vi "Robotic Arm controler.vi"(1 "write?":bool, 2 "Servo angle":dbl(knob)=90.0 scale=0.0..180.0, 3 "Servo number":i32(knob)=3 scale=1.0..6.0) -> (0 "Command to robotic arm":string)   [LabVIEW 2015]
doc: "Sends the commands to the Robotic Arm based on the servo number and angle provided as the inputs."
uses:
  <vilib>/Instr/_visa.llb/VISA Configure Serial Port (Instr).vi
panel:
  # "Servo number"
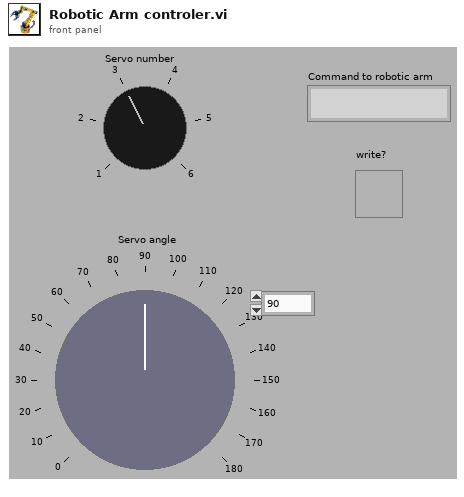
[diagram p1: front panel]
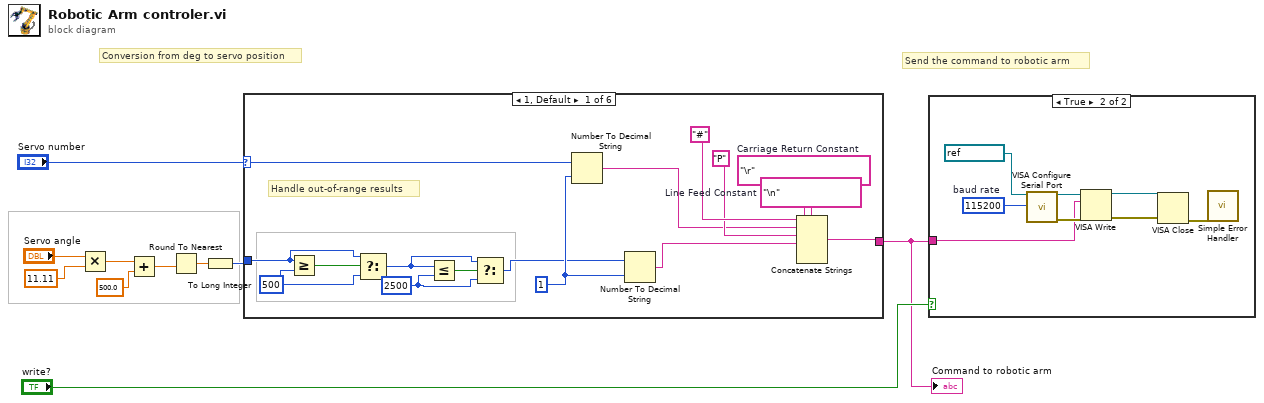
[diagram p0: block diagram]
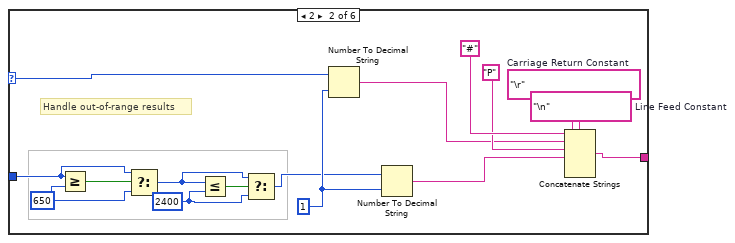
[diagram p3: hidden frame]
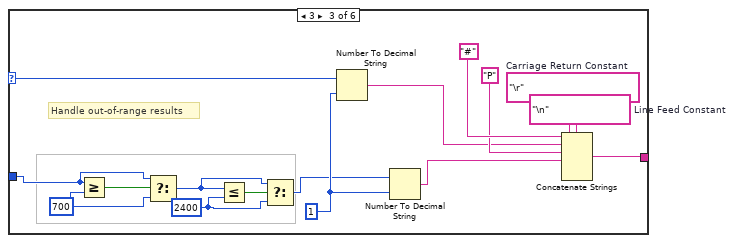
[diagram p4: hidden frame]
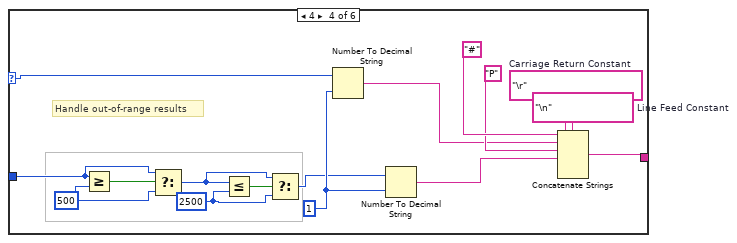
[diagram p5: hidden frame]
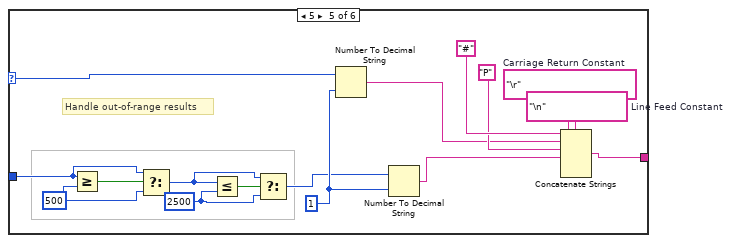
[diagram p6: hidden frame]
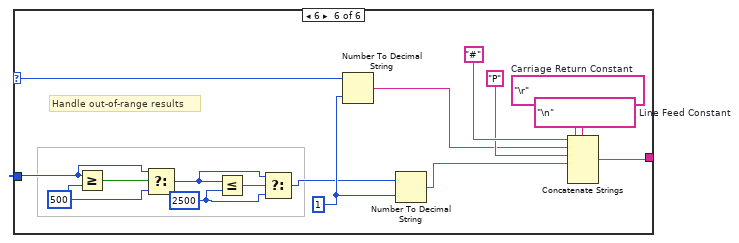
[diagram p7: hidden frame]
diagram:
  # "Send the command to robotic arm"
  # "Conversion from deg to servo position"
  n1 = Multiply(x="Servo angle", y=11.11) -> (x*y=w5:dbl)
  n2 = Add(x=w5, y=500.0) -> (x+y=w4:dbl)
  n3 = Round To Nearest(number=w4) -> (nearest integer value=w2:dbl)
  n4 = To Long Integer(number=w2) -> (32bit integer=w1:i32)
  n5 = case shown="1, Default" "Servo number" {
    selector: "Servo number" -> [w25 w35 w51 w67 w83 w99]
    tunnel: [w20 w34 w50 w66 w82 w98] -> w9
    tunnel: w1 -> [w15 w28 w44 w60 w76 w92]
    frame 1, Default {
      w13 = 2500 ("y")
      w16 = 500 ("y")
      w22 = "\r"  # Carriage Return Constant
      w21 = "\n"  # Line Feed Constant
      w26 = i16 1 ("width (-)")
      # "Handle out-of-range results"
      n6 = Greater Or Equal?(x=w15, y=w16) -> (x >= y?=w17:bool)
      n7 = Select(t=w15, s=w17, f=w16) -> (s? t:f=w12:i32)
      n8 = Less Or Equal?(x=w12, y=w13) -> (x <= y?=w14:bool)
      n9 = Select(t=w12, s=w14, f=w13) -> (s? t:f=w11:i32)
      n10 = Number To Decimal String(number=w25, width (-)=w26) -> (decimal integer string=w18:string)
      n11 = Number To Decimal String(number=w11, width (-)=w26) -> (decimal integer string=w19:string)
      n12 = Concatenate Strings "Concatenate Strings"("#" ("string"), w18, "P" ("string"), w19, w22, w21) -> (w20:string)
    }
    frame 2 {
      w30 = 2400 ("y")
      w32 = 650 ("y")
      w39 = "\r"  # Carriage Return Constant
      w38 = "\n"  # Line Feed Constant
      w42 = i16 1 ("width (-)")
      # "Handle out-of-range results"
      n13 = Greater Or Equal?(x=w28, y=w32) -> (x >= y?=w33:bool)
      n14 = Select(t=w28, s=w33, f=w32) -> (s? t:f=w29:i32)
      n15 = Less Or Equal?(x=w29, y=w30) -> (x <= y?=w31:bool)
      n16 = Select(t=w29, s=w31, f=w30) -> (s? t:f=w27:i32)
      n17 = Number To Decimal String(number=w35, width (-)=w42) -> (decimal integer string=w36:string)
      n18 = Number To Decimal String(number=w27, width (-)=w42) -> (decimal integer string=w37:string)
      n19 = Concatenate Strings "Concatenate Strings"("#" ("string"), w36, "P" ("string"), w37, w39, w38) -> (w34:string)
    }
    frame 3 {
      w46 = 2400 ("y")
      w48 = 700 ("y")
      w55 = "\r"  # Carriage Return Constant
      w54 = "\n"  # Line Feed Constant
      w58 = i16 1 ("width (-)")
      # "Handle out-of-range results"
      n20 = Greater Or Equal?(x=w44, y=w48) -> (x >= y?=w49:bool)
      n21 = Select(t=w44, s=w49, f=w48) -> (s? t:f=w45:i32)
      n22 = Less Or Equal?(x=w45, y=w46) -> (x <= y?=w47:bool)
      n23 = Select(t=w45, s=w47, f=w46) -> (s? t:f=w43:i32)
      n24 = Number To Decimal String(number=w51, width (-)=w58) -> (decimal integer string=w52:string)
      n25 = Number To Decimal String(number=w43, width (-)=w58) -> (decimal integer string=w53:string)
      n26 = Concatenate Strings "Concatenate Strings"("#" ("string"), w52, "P" ("string"), w53, w55, w54) -> (w50:string)
    }
    frame 4 {
      w62 = 2500 ("y")
      w64 = 500 ("y")
      w71 = "\r"  # Carriage Return Constant
      w70 = "\n"  # Line Feed Constant
      w74 = i16 1 ("width (-)")
      # "Handle out-of-range results"
      n27 = Greater Or Equal?(x=w60, y=w64) -> (x >= y?=w65:bool)
      n28 = Select(t=w60, s=w65, f=w64) -> (s? t:f=w61:i32)
      n29 = Less Or Equal?(x=w61, y=w62) -> (x <= y?=w63:bool)
      n30 = Select(t=w61, s=w63, f=w62) -> (s? t:f=w59:i32)
      n31 = Number To Decimal String(number=w67, width (-)=w74) -> (decimal integer string=w68:string)
      n32 = Number To Decimal String(number=w59, width (-)=w74) -> (decimal integer string=w69:string)
      n33 = Concatenate Strings "Concatenate Strings"("#" ("string"), w68, "P" ("string"), w69, w71, w70) -> (w66:string)
    }
    frame 5 {
      w78 = 2500 ("y")
      w80 = 500 ("y")
      w87 = "\r"  # Carriage Return Constant
      w86 = "\n"  # Line Feed Constant
      w90 = i16 1 ("width (-)")
      # "Handle out-of-range results"
      n34 = Greater Or Equal?(x=w76, y=w80) -> (x >= y?=w81:bool)
      n35 = Select(t=w76, s=w81, f=w80) -> (s? t:f=w77:i32)
      n36 = Less Or Equal?(x=w77, y=w78) -> (x <= y?=w79:bool)
      n37 = Select(t=w77, s=w79, f=w78) -> (s? t:f=w75:i32)
      n38 = Number To Decimal String(number=w83, width (-)=w90) -> (decimal integer string=w84:string)
      n39 = Number To Decimal String(number=w75, width (-)=w90) -> (decimal integer string=w85:string)
      n40 = Concatenate Strings "Concatenate Strings"("#" ("string"), w84, "P" ("string"), w85, w87, w86) -> (w82:string)
    }
    frame 6 {
      w94 = 2500 ("y")
      w96 = 500 ("y")
      w103 = "\r"  # Carriage Return Constant
      w102 = "\n"  # Line Feed Constant
      w106 = i16 1 ("width (-)")
      # "Handle out-of-range results"
      n41 = Greater Or Equal?(x=w92, y=w96) -> (x >= y?=w97:bool)
      n42 = Select(t=w92, s=w97, f=w96) -> (s? t:f=w93:i32)
      n43 = Less Or Equal?(x=w93, y=w94) -> (x <= y?=w95:bool)
      n44 = Select(t=w93, s=w95, f=w94) -> (s? t:f=w91:i32)
      n45 = Number To Decimal String(number=w99, width (-)=w106) -> (decimal integer string=w100:string)
      n46 = Number To Decimal String(number=w91, width (-)=w106) -> (decimal integer string=w101:string)
      n47 = Concatenate Strings "Concatenate Strings"("#" ("string"), w100, "P" ("string"), w101, w103, w102) -> (w98:string)
    }
  }
  "Command to robotic arm" <- w9
  n48 = case shown="True" "write?" {
    tunnel: w9 -> [_ w111]
    frame False {
    }
    frame True {
      w114 = u32 115200  # baud rate
      n49 = call-poly "VISA Configure Serial Port"("VISA resource name"=refnum<visa-resource-name> "COM4", "baud rate (9600)"=w114) -> ("VISA resource name out"=w112:refnum<visa-resource-name>, "error out"=w113:errorcluster)  [unwired: 7 in, 5 out]
      n50 = VISA Write(VISA resource name=w112, write buffer=w111, error in (no error)=w113) -> (VISA resource name out=w108:refnum<visa-resource-name>, error out=w107:errorcluster)  [unwired: 1 out]
      n51 = VISA Close(VISA resource name=w108, error in (no error)=w107) -> (error out=w110:errorcluster)
      n52 = call <vilib>:"Simple Error Handler.vi"("error in (no error)"=w110) -> ()  [unwired: 1 in, 8 out]
    }
  }
